vi "报表.vi"() -> ()   [LabVIEW 2018]
uses:
  <vilib>/Utility/NIReport.llb/Report Type.ctl
  <vilib>/Utility/NIReport.llb/Append Report Text (str wrap).vi
  <vilib>/addons/_office/word.llb/Word Edit Cell ([dbl]).vi
  <vilib>/Utility/NIReport.llb/NI_report.lvclass
  <vilib>/Utility/NIReport.llb/Word/NI_Word.lvclass
  <vilib>/addons/_office/NI_ReportGenerationToolkit.lvlib
  <vilib>/Utility/NIReport.llb/NI_ReportGenerationCore.lvlib
panel:
  out "报表进度":dbl
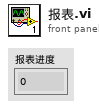
[diagram p1: front panel]
types:
  T1 = cluster{"position (Excel)":cluster{"row":i32, "column":i32}, "name (Excel)":string, "bookmark (Word)":string}
  T2 = typedef "NI_ReportGenerationCore.lvlib/Report Type.ctl" = enum16{"HTML", "Word", "Excel"}
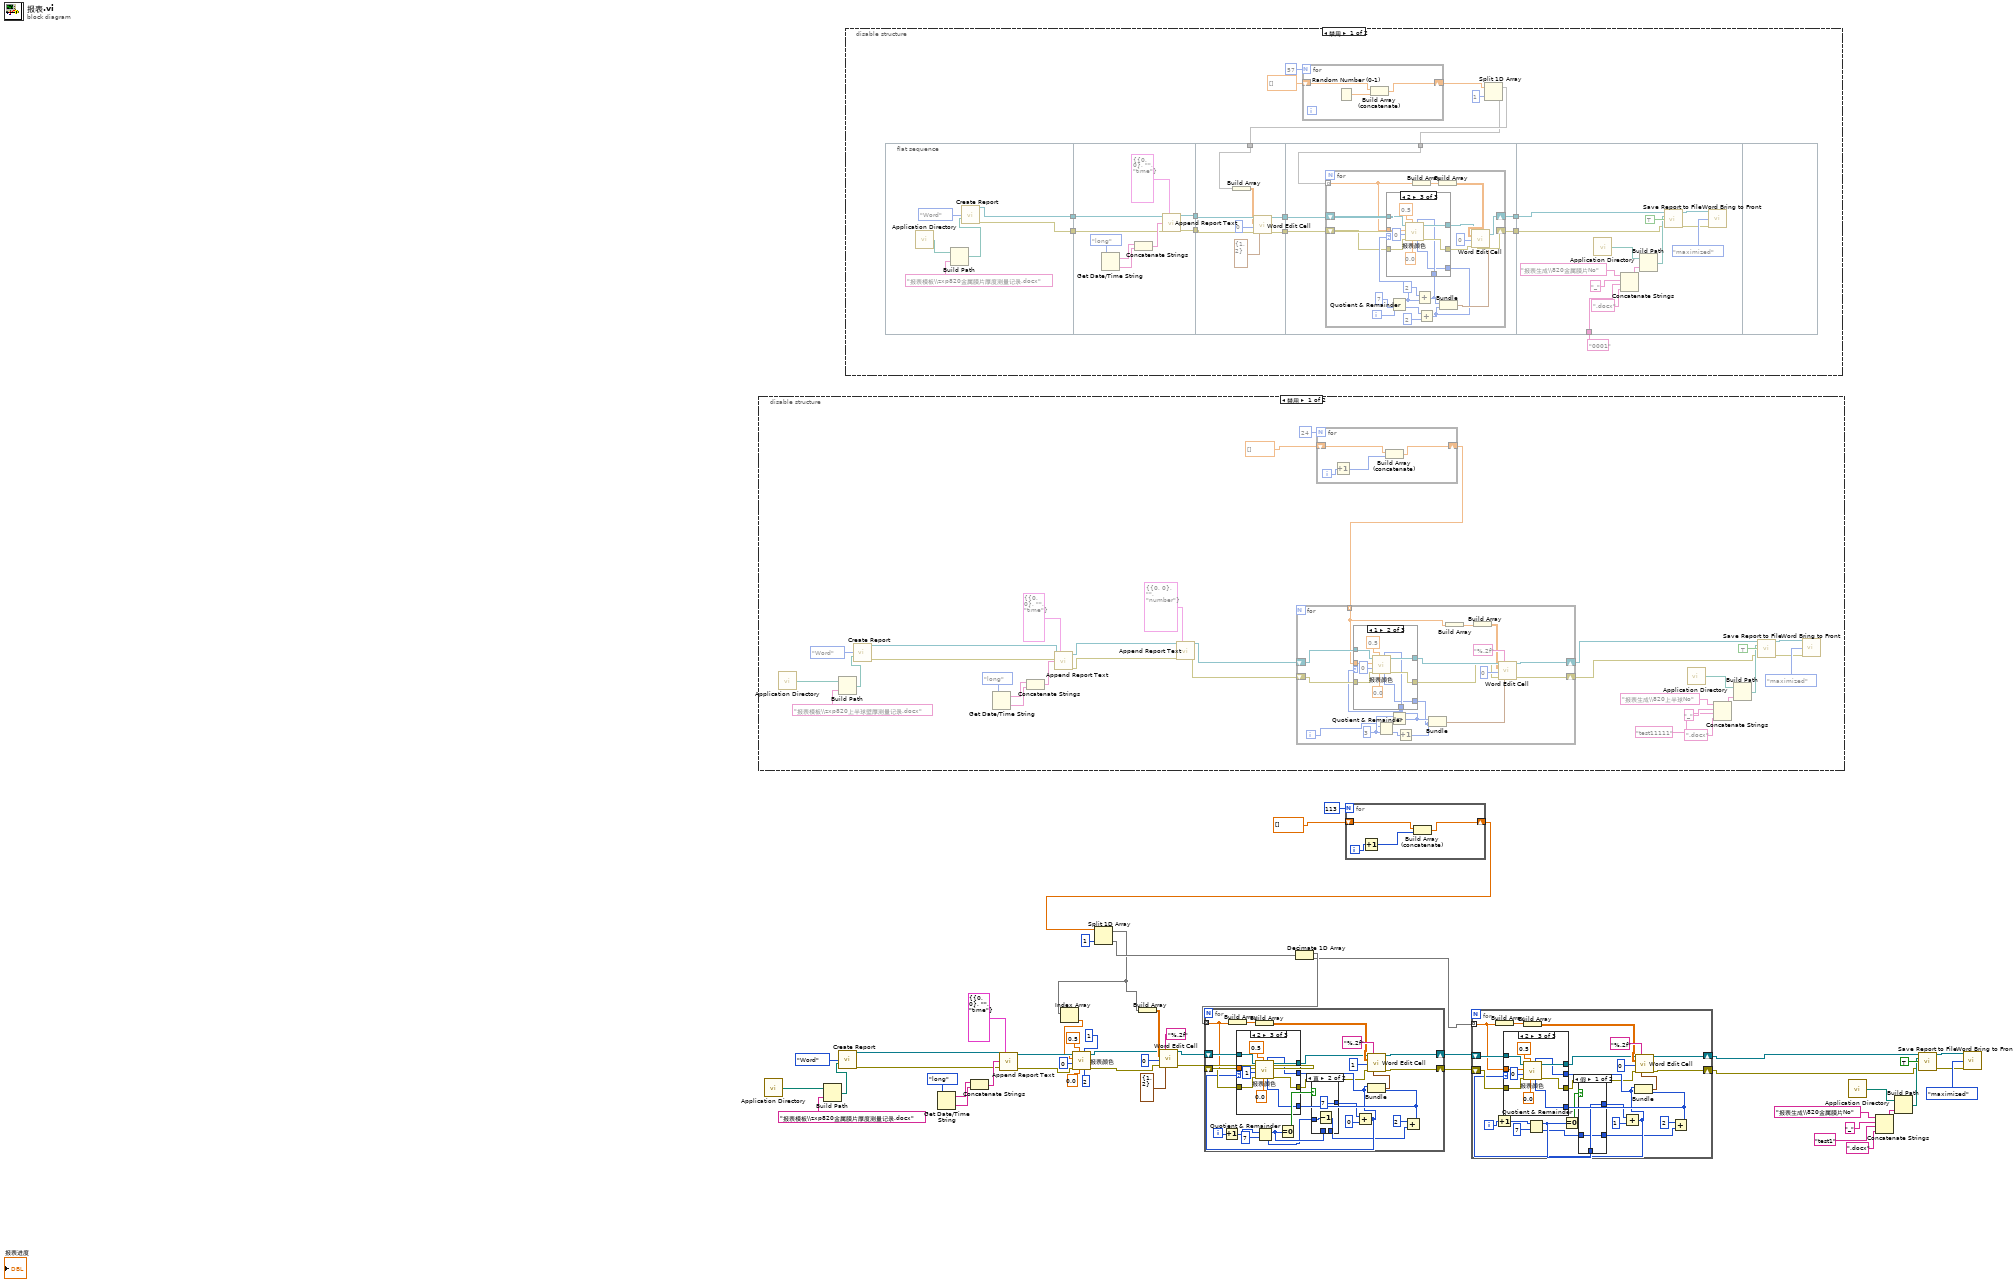
[diagram p0: block diagram]
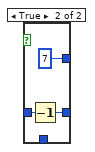
[diagram p2: hidden frame]
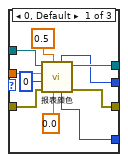
[diagram p3: hidden frame]
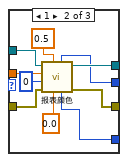
[diagram p4: hidden frame]
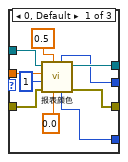
[diagram p6: hidden frame]
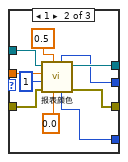
[diagram p7: hidden frame]
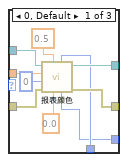
[diagram p8: hidden frame]
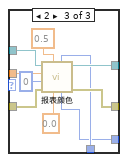
[diagram p9: hidden frame]
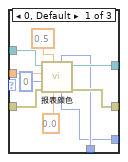
[diagram p11: hidden frame]
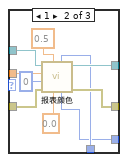
[diagram p12: hidden frame]
diagram:
  n1 = disable-structure shown="禁用" {
    frame Disabled {
      n2 = call <vilib>:"Application Directory.vi"() -> ("Application Directory"=w80:path)
      n3 = Build Path(base path=w80, name or relative path="报表模板\\zxp820上半球壁厚测量记录.docx") -> (appended path=w77:path)
      n4 = call <vilib>:"Create Report.vi"("report type"=Report_Type."Word" ("Report Type"), "template (empty)"=w77) -> ("report out"=w61:refnum<class "NI_report.lvclass">, "error out"=w60:errorcluster)  [unwired: 12 in]
      n5 = Get Date/Time String(date format (0)=enum16{"short", "long", "abbreviated"}."long" ("日期格式(0)")) -> (date string=w76:string, time string=w74:string)  [unwired: 2 in]
      n6 = Concatenate Strings(w76, w74) -> (w75:string)
      n7 = call-poly <vilib>:"Append Report Text.vi"("report in"=w61, "MS Office parameters"=T1 {"position (Excel)"={"row"=0, "column"=0}, "name (Excel)"="", "bookmark (Word)"="time"}, "text"=w75, "error in (no error)"=w60) -> ("report out"=w58:refnum<class "NI_report.lvclass">, "error out"=w57:errorcluster)  [unwired: 8 in, 2 out]
      n8 = call-poly <vilib>:"Append Report Text.vi"("report in"=w58, "MS Office parameters"=T1 {"position (Excel)"={"row"=0, "column"=0}, "name (Excel)"="", "bookmark (Word)"="number"}, "error in (no error)"=w57) -> ("report out"=w56:refnum<class "NI_report.lvclass">, "error out"=w55:errorcluster)  [unwired: 9 in, 2 out]
      n9 = for {
        N: 24 -> [_]
        shift-right: [w133] -> w52
        shift-left: dbl[] [] -> [w134]
        i -> [w132]
        n10 = Increment(x=w132) -> (x+1=w131:i32)
        n11 = Build Array (concatenate)(w134, w131) -> (w133:dbl[])
      }
      n12 = for {
        shift-right: [w99] -> w54
        shift-left: w56 -> [w96]
        shift-right: [w98] -> w53
        shift-left: w55 -> [w95]
        tunnel: w52 -> [w92] mode=indexing
        i -> [w83]
        w87 = 3 ("y")
        n13 = Quotient & Remainder(x=w83, y=w87) -> (x-y*floor(x/y)=w88:i32, floor(x/y)=w85:i32)
        n14 = Subtract(x=w87, y=w88) -> (x-y=w86:i32)
        n15 = Increment(x=w85) -> (x+1=w84:i32)
        n16 = case shown="1" w86 {
          tunnel: w96 -> [w110 w120 w130]
          tunnel: [w109 w119 w129] -> w94
          tunnel: [w108 w118 w128] -> w93
          tunnel: w95 -> [w107 w117 w127]
          tunnel: w92 -> [w104 w114 w124]
          tunnel: w86 -> [w103 w113 w123]
          tunnel: w84 -> [w102 w112 w122]
          frame 0, Default {
            n17 = call "报表颜色.vi"("列"=w102, "行"=w103, "下限"=0.0, "上限"=0.5, "error in (no error)"=w107, "table index (-1)"=i16 0, "厚度值"=w104, "report in"=w110) -> ("error out"=w108:errorcluster, "report out"=w109:refnum<class "NI_report.lvclass">)  [unwired: 2 in]
          }
          frame 1 {
            n18 = call "报表颜色.vi"("列"=w112, "行"=w113, "下限"=0.0, "上限"=0.5, "error in (no error)"=w117, "table index (-1)"=i16 0, "厚度值"=w114, "report in"=w120) -> ("error out"=w118:errorcluster, "report out"=w119:refnum<class "NI_report.lvclass">)  [unwired: 2 in]
          }
          frame 2 {
            n19 = call "报表颜色.vi"("列"=w122, "行"=w123, "下限"=0.0, "上限"=0.5, "error in (no error)"=w127, "table index (-1)"=i16 0, "厚度值"=w124, "report in"=w130) -> ("error out"=w128:errorcluster, "report out"=w129:refnum<class "NI_report.lvclass">)  [unwired: 2 in]
          }
        }
        n20 = Bundle(w86, w84) -> (w89:cluster{i32, i32})  [unwired: 1 in]
        n21 = Build Array(w92) -> (w91:dbl[])
        n22 = Build Array(w91) -> (w90:dbl[][])
        n23 = call-poly <vilib>:"Word Edit Cell.vi"("report in"=w94, "format string (%.3f)"="%.2f", "value"=w90, "table index (-1)"=i16 0, "error in (no error)"=w93, "start (0, 0)"=w89) -> ("report out"=w99:refnum<class "NI_report.lvclass">, "error out"=w98:errorcluster)  [unwired: 8 in]
      }
      n24 = call <vilib>:"Application Directory.vi"() -> ("Application Directory"=w69:path)
      n25 = Concatenate Strings("报表生成\\820上半球No" ("字符串"), "_" ("名称或相对路径"), "test11111" ("字符串"), ".docx" ("名称或相对路径")) -> (w68:string)
      n26 = Build Path(base path=w69, name or relative path=w68) -> (appended path=w70:path)
      n27 = call-dynamic "Save Report to File.vi"("report in"=w54, "report file path"=w70, "prompt to replace? (F)"=TRUE, "error in (no error)"=w53) -> ("report out"=w63:refnum<class "NI_report.lvclass">, "error out"=w62:errorcluster)  [unwired: 10 in]
      n28 = call <vilib>:"Word Bring to Front.vi"("report in"=w63, "window state (maximized)"=enum16{"maximized", "minimized", "normal"}."maximized", "error in (no error)"=w62) -> ()  [unwired: 11 in, 2 out]
    }
    frame Enabled {
    }
  }
  n29 = call <vilib>:"Application Directory.vi"() -> ("Application Directory"=w45:path)
  n30 = Build Path(base path=w45, name or relative path="报表模板\\zxp820金属膜片厚度测量记录.docx") -> (appended path=w42:path)
  n31 = call <vilib>:"Create Report.vi"("report type"=Report_Type."Word" ("Report Type"), "template (empty)"=w42) -> ("report out"=w22:refnum<class "NI_report.lvclass">, "error out"=w21:errorcluster)  [unwired: 12 in]
  n32 = disable-structure shown="禁用" {
    frame Disabled {
      n33 = flat-sequence {
        tunnel: [w151] -> w149
        tunnel: [w150] -> w148
        tunnel: [w159] -> w147
        tunnel: [w158] -> w146
        tunnel: w149 -> [w157]
        tunnel: w148 -> [w156]
        tunnel: w147 -> [w170]
        tunnel: w146 -> [w169]
        tunnel: [w168] -> w145
        tunnel: [w167] -> w144
        tunnel: w138 -> [w166]
        tunnel: w145 -> [w177]
        tunnel: w144 -> [w176]
        tunnel: w137 -> [w173]
        tunnel: [w175] -> w143
        tunnel: [w174] -> w142
        tunnel: w143 -> [w231]
        tunnel: w142 -> [w230]
        tunnel: "0001" ("工件编号：") -> [w233]
        frame #0 {
          n34 = call <vilib>:"Application Directory.vi"() -> ("Application Directory"=w154:path)
          n35 = Build Path(base path=w154, name or relative path="报表模板\\zxp820金属膜片厚度测量记录.docx") -> (appended path=w152:path)
          n36 = call <vilib>:"Create Report.vi"("report type"=Report_Type."Word" ("Report Type"), "template (empty)"=w152) -> ("report out"=w151:refnum<class "NI_report.lvclass">, "error out"=w150:errorcluster)  [unwired: 12 in]
        }
        frame #1 {
          n37 = Get Date/Time String(date format (0)=enum16{"short", "long", "abbreviated"}."long" ("日期格式(0)")) -> (date string=w164:string, time string=w162:string)  [unwired: 2 in]
          n38 = Concatenate Strings(w164, w162) -> (w163:string)
          n39 = call-poly <vilib>:"Append Report Text.vi"("report in"=w157, "MS Office parameters"=T1 {"position (Excel)"={"row"=0, "column"=0}, "name (Excel)"="", "bookmark (Word)"="time"}, "text"=w163, "error in (no error)"=w156) -> ("report out"=w159:refnum<class "NI_report.lvclass">, "error out"=w158:errorcluster)  [unwired: 8 in, 2 out]
        }
        frame #2 {
          n40 = Build Array(w166) -> (w165:dbl[][])
          n41 = call-poly <vilib>:"Word Edit Cell.vi"("report in"=w170, "value"=w165, "table index (-1)"=i16 0, "error in (no error)"=w169, "start (0, 0)"=cluster{"row":i32, "column":i32} {"row"=1, "column"=2}) -> ("report out"=w168:refnum<class "NI_report.lvclass">, "error out"=w167:errorcluster)  [unwired: 9 in]
        }
        frame #3 {
          n42 = for {
            shift-right: [w195] -> w175
            shift-left: w177 -> [w181]
            shift-right: [w194] -> w174
            shift-left: w176 -> [w180]
            tunnel: w173 -> [w182] mode=indexing
            i -> [w190]
            n43 = Quotient & Remainder(x=w190, y=7) -> (x-y*floor(x/y)=w185:i32, floor(x/y)=w187:i32)
            n44 = Build Array(w182) -> (w192:dbl[])
            n45 = Add(x=2 ("索引"), y=w185) -> (x+y=w179:i32)
            n46 = Add(x=w187, y=2) -> (x+y=w178:i32)
            n47 = case shown="2" w185 {
              tunnel: w181 -> [w206 w216 w226]
              tunnel: [w205 w215 w225] -> w184
              tunnel: [w204 w214 w224] -> w183
              tunnel: w180 -> [w203 w213 w223]
              tunnel: w182 -> [w200 w210 w220]
              tunnel: w179 -> [w199 w209 w219]
              tunnel: w178 -> [w198 w208 w218]
              frame 0, Default {
                n48 = call "报表颜色.vi"("列"=w198, "行"=w199, "下限"=0.0, "上限"=0.5, "error in (no error)"=w203, "table index (-1)"=i16 0, "厚度值"=w200, "report in"=w206) -> ("error out"=w204:errorcluster, "report out"=w205:refnum<class "NI_report.lvclass">)  [unwired: 2 in]
              }
              frame 1 {
                n49 = call "报表颜色.vi"("列"=w208, "行"=w209, "下限"=0.0, "上限"=0.5, "error in (no error)"=w213, "table index (-1)"=i16 0, "厚度值"=w210, "report in"=w216) -> ("error out"=w214:errorcluster, "report out"=w215:refnum<class "NI_report.lvclass">)  [unwired: 2 in]
              }
              frame 2 {
                n50 = call "报表颜色.vi"("列"=w218, "行"=w219, "下限"=0.0, "上限"=0.5, "error in (no error)"=w223, "table index (-1)"=i16 0, "厚度值"=w220, "report in"=w226) -> ("error out"=w224:errorcluster, "report out"=w225:refnum<class "NI_report.lvclass">)  [unwired: 2 in]
              }
            }
            n51 = Build Array(w192) -> (w191:dbl[][])
            n52 = Bundle(w179, w178) -> (w193:cluster{i32, i32})  [unwired: 1 in]
            n53 = call-poly <vilib>:"Word Edit Cell.vi"("report in"=w184, "value"=w191, "table index (-1)"=i16 0, "error in (no error)"=w183, "start (0, 0)"=w193) -> ("report out"=w195:refnum<class "NI_report.lvclass">, "error out"=w194:errorcluster)  [unwired: 9 in]
          }
        }
        frame #4 {
          n54 = call <vilib>:"Application Directory.vi"() -> ("Application Directory"=w237:path)
          n55 = Concatenate Strings("报表生成\\820金属膜片No" ("字符串"), "_" ("名称或相对路径"), w233, ".docx" ("名称或相对路径")) -> (w236:string)
          n56 = Build Path(base path=w237, name or relative path=w236) -> (appended path=w238:path)
          n57 = call-dynamic "Save Report to File.vi"("report in"=w231, "report file path"=w238, "prompt to replace? (F)"=TRUE, "error in (no error)"=w230) -> ("report out"=w228:refnum<class "NI_report.lvclass">, "error out"=w227:errorcluster)  [unwired: 10 in]
          n58 = call <vilib>:"Word Bring to Front.vi"("report in"=w228, "window state (maximized)"=enum16{"maximized", "minimized", "normal"}."maximized", "error in (no error)"=w227) -> ()  [unwired: 11 in, 2 out]
        }
        frame #5 {
        }
      }
      n59 = for {
        N: 57 -> [_]
        shift-right: [w240] -> w139
        shift-left: dbl[] [] -> [w241]
        n60 = Random Number (0-1)() -> (number: 0 to 1=w242:dbl)
        n61 = Build Array (concatenate)(w241, w242) -> (w240:dbl[])
      }
      n62 = Split 1D Array(array=w139, index=1 ("索引")) -> (first subarray=w138:dbl[], second subarray=w137:dbl[])
    }
    frame Enabled {
    }
  }
  n63 = Get Date/Time String(date format (0)=enum16{"short", "long", "abbreviated"}."long" ("日期格式(0)")) -> (date string=w41:string, time string=w39:string)  [unwired: 2 in]
  n64 = Concatenate Strings(w41, w39) -> (w40:string)
  n65 = call-poly <vilib>:"Append Report Text.vi"("report in"=w22, "MS Office parameters"=T1 {"position (Excel)"={"row"=0, "column"=0}, "name (Excel)"="", "bookmark (Word)"="time"}, "text"=w40, "error in (no error)"=w21) -> ("report out"=w17:refnum<class "NI_report.lvclass">, "error out"=w16:errorcluster)  [unwired: 8 in, 2 out]
  n66 = for {
    N: 113 -> [_]
    shift-right: [w245] -> w2
    shift-left: dbl[] [] -> [w246]
    i -> [w244]
    n67 = Increment(x=w244) -> (x+1=w243:i32)
    n68 = Build Array (concatenate)(w246, w243) -> (w245:dbl[])
  }
  n69 = Split 1D Array(array=w2, index=1 ("索引")) -> (first subarray=w13:dbl[], second subarray=w46:dbl[])
  n70 = Index Array(array=w13) -> (element=w12:dbl)  [unwired: 1 in]
  n71 = call "报表颜色.vi"("列"=i8 2, "行"=i8 1, "下限"=0.0, "上限"=0.5, "error in (no error)"=w16, "table index (-1)"=i16 0, "厚度值"=w12, "report in"=w17) -> ("error out"=w10:errorcluster, "report out"=w11:refnum<class "NI_report.lvclass">)  [unwired: 2 in]
  n72 = Build Array(w13) -> (w34:dbl[][])
  n73 = call-poly <vilib>:"Word Edit Cell.vi"("report in"=w11, "format string (%.3f)"="%.2f", "value"=w34, "table index (-1)"=i16 0, "error in (no error)"=w10, "start (0, 0)"=cluster{"row":i32, "column":i32} {"row"=1, "column"=2}) -> ("report out"=w9:refnum<class "NI_report.lvclass">, "error out"=w47:errorcluster)  [unwired: 8 in]
  n74 = Decimate 1D Array(w46) -> (w8:dbl[], w7:dbl[])
  n75 = for {
    shift-right: [w269] -> w6
    shift-left: w9 -> [w263]
    shift-right: [w268] -> w5
    shift-left: w47 -> [w262]
    tunnel: w8 -> [w261] mode=indexing
    i -> [w253]
    n76 = Increment(x=w253) -> (x+1=w252:i32)
    n77 = Build Array(w261) -> (w265:dbl[])
    n78 = Build Array(w265) -> (w264:dbl[][])
    n79 = Quotient & Remainder(x=w252, y=7) -> (x-y*floor(x/y)=w254:i32, floor(x/y)=w248:i32)
    n80 = Equal To 0?(x=w254) -> (x = 0?=w257:bool)
    n81 = case shown="真" w257 {
      tunnel: [w272 7 ("y")] -> w255
      tunnel: w254 -> [w272 _]
      tunnel: w248 -> [w271 w274]
      tunnel: [w271 w273] -> w247
      frame False {
      }
      frame True {
        n82 = Decrement(x=w274) -> (x-1=w273:i32)
      }
    }
    n83 = Add(x=w255, y=0 ("x")) -> (x+y=w251:i32)
    n84 = Add(x=2, y=w247) -> (x+y=w258:i32)
    n85 = case shown="2" w251 {
      tunnel: w263 -> [w285 w295 w305]
      tunnel: [w284 w294 w304] -> w250
      tunnel: [w283 w293 w303] -> w249
      tunnel: w262 -> [w282 w292 w302]
      tunnel: w261 -> [w279 w289 w299]
      tunnel: w258 -> [w278 w288 w298]
      tunnel: w251 -> [w276 w286 w296]
      frame 0, Default {
        n86 = call "报表颜色.vi"("列"=w278, "行"=w276, "下限"=0.0, "上限"=0.5, "error in (no error)"=w282, "table index (-1)"=i16 1, "厚度值"=w279, "report in"=w285) -> ("error out"=w283:errorcluster, "report out"=w284:refnum<class "NI_report.lvclass">)  [unwired: 2 in]
      }
      frame 1 {
        n87 = call "报表颜色.vi"("列"=w288, "行"=w286, "下限"=0.0, "上限"=0.5, "error in (no error)"=w292, "table index (-1)"=i16 1, "厚度值"=w289, "report in"=w295) -> ("error out"=w293:errorcluster, "report out"=w294:refnum<class "NI_report.lvclass">)  [unwired: 2 in]
      }
      frame 2 {
        n88 = call "报表颜色.vi"("列"=w298, "行"=w296, "下限"=0.0, "上限"=0.5, "error in (no error)"=w302, "table index (-1)"=i16 1, "厚度值"=w299, "report in"=w305) -> ("error out"=w303:errorcluster, "report out"=w304:refnum<class "NI_report.lvclass">)  [unwired: 2 in]
      }
    }
    n89 = Bundle(w251, w258) -> (w267:cluster{i32, i32})  [unwired: 1 in]
    n90 = call-poly <vilib>:"Word Edit Cell.vi"("report in"=w250, "format string (%.3f)"="%.2f", "value"=w264, "table index (-1)"=i16 1, "error in (no error)"=w249, "start (0, 0)"=w267) -> ("report out"=w269:refnum<class "NI_report.lvclass">, "error out"=w268:errorcluster)  [unwired: 8 in]
  }
  n91 = for {
    shift-right: [w328] -> w4
    shift-left: w6 -> [w322]
    shift-right: [w327] -> w3
    shift-left: w5 -> [w321]
    tunnel: w7 -> [w320] mode=indexing
    i -> [w312]
    n92 = Increment(x=w312) -> (x+1=w311:i32)
    n93 = Build Array(w320) -> (w324:dbl[])
    n94 = Build Array(w324) -> (w323:dbl[][])
    n95 = Quotient & Remainder(x=w311, y=7) -> (x-y*floor(x/y)=w313:i32, floor(x/y)=w307:i32)
    n96 = Equal To 0?(x=w313) -> (x = 0?=w316:bool)
    n97 = case shown="假" w316 {
      tunnel: [w331 7 ("y")] -> w314
      tunnel: w313 -> [w331 _]
      tunnel: w307 -> [w330 w333]
      tunnel: [w330 w332] -> w306
      frame False {
      }
      frame True {
        n98 = Decrement(x=w333) -> (x-1=w332:i32)
      }
    }
    n99 = Add(x=w314, y=1 ("x")) -> (x+y=w310:i32)
    n100 = Add(x=2, y=w306) -> (x+y=w317:i32)
    n101 = case shown="2" w310 {
      tunnel: w322 -> [w344 w354 w364]
      tunnel: [w343 w353 w363] -> w309
      tunnel: [w342 w352 w362] -> w308
      tunnel: w321 -> [w341 w351 w361]
      tunnel: w320 -> [w338 w348 w358]
      tunnel: w317 -> [w337 w347 w357]
      tunnel: w310 -> [w335 w345 w355]
      frame 0, Default {
        n102 = call "报表颜色.vi"("列"=w337, "行"=w335, "下限"=0.0, "上限"=0.5, "error in (no error)"=w341, "table index (-1)"=i16 0, "厚度值"=w338, "report in"=w344) -> ("error out"=w342:errorcluster, "report out"=w343:refnum<class "NI_report.lvclass">)  [unwired: 2 in]
      }
      frame 1 {
        n103 = call "报表颜色.vi"("列"=w347, "行"=w345, "下限"=0.0, "上限"=0.5, "error in (no error)"=w351, "table index (-1)"=i16 0, "厚度值"=w348, "report in"=w354) -> ("error out"=w352:errorcluster, "report out"=w353:refnum<class "NI_report.lvclass">)  [unwired: 2 in]
      }
      frame 2 {
        n104 = call "报表颜色.vi"("列"=w357, "行"=w355, "下限"=0.0, "上限"=0.5, "error in (no error)"=w361, "table index (-1)"=i16 0, "厚度值"=w358, "report in"=w364) -> ("error out"=w362:errorcluster, "report out"=w363:refnum<class "NI_report.lvclass">)  [unwired: 2 in]
      }
    }
    n105 = Bundle(w310, w317) -> (w326:cluster{i32, i32})  [unwired: 1 in]
    n106 = call-poly <vilib>:"Word Edit Cell.vi"("report in"=w309, "format string (%.3f)"="%.2f", "value"=w323, "table index (-1)"=i16 0, "error in (no error)"=w308, "start (0, 0)"=w326) -> ("report out"=w328:refnum<class "NI_report.lvclass">, "error out"=w327:errorcluster)  [unwired: 8 in]
  }
  n107 = call <vilib>:"Application Directory.vi"() -> ("Application Directory"=w30:path)
  n108 = Concatenate Strings("报表生成\\820金属膜片No" ("字符串"), "_" ("名称或相对路径"), "test1" ("名称或相对路径"), ".docx" ("名称或相对路径")) -> (w29:string)
  n109 = Build Path(base path=w30, name or relative path=w29) -> (appended path=w31:path)
  n110 = call-dynamic "Save Report to File.vi"("report in"=w4, "report file path"=w31, "prompt to replace? (F)"=TRUE, "error in (no error)"=w3) -> ("report out"=w24:refnum<class "NI_report.lvclass">, "error out"=w23:errorcluster)  [unwired: 10 in]
  n111 = call <vilib>:"Word Bring to Front.vi"("report in"=w24, "window state (maximized)"=enum16{"maximized", "minimized", "normal"}."maximized", "error in (no error)"=w23) -> ()  [unwired: 11 in, 2 out]
